vi "Check_Range_Vals.vi"(1 "Increment":dbl, 2 "Lower Limit":dbl, 3 "Upper Limit":dbl) -> (0 "Bounds Are Good":bool)   [LabVIEW 2019]
doc: "Given initial and final positions with an increment are all the values ordered correctly? \n\ni.e. is final > initial and is final - initial > increment? \n\nR. Sheehan 21 - 4 - 2015"
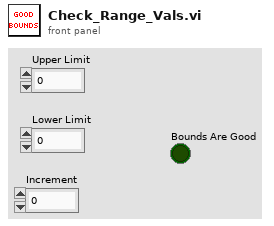
[diagram p1: front panel]
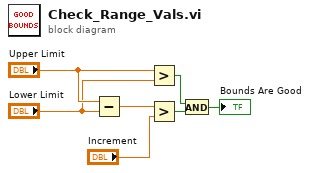
[diagram p0: block diagram]
diagram:
  n1 = Subtract(x="Upper Limit", y="Lower Limit") -> (x-y=w5:dbl)
  n2 = Greater?(x="Upper Limit", y="Lower Limit") -> (0:w3:bool)
  n3 = Greater?(x=w5, y="Increment") -> (0:w2:bool)
  n4 = And(x=w3, y=w2) -> (x .and. y?=→"Bounds Are Good":bool)
